vi "CN Config Panel.vi"(8 "error in":errorcluster, 11 "Path":path) -> (0 "error out":errorcluster)   [LabVIEW 2014]
uses:
  Type'def/CN Config Ctr.ctl
panel:
  in  "Exit":bool
  in  "Save Data":bool
  in  "CN Configs":T1[](array[typedef])
  # "Customer Information Config"
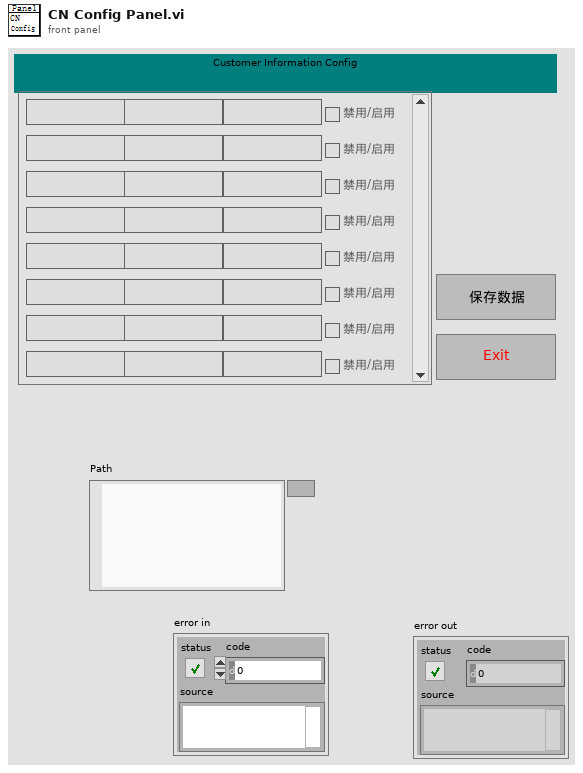
[diagram p1: front panel]
types:
  T1 = typedef "CN Config Ctr.ctl" = cluster{"Model":string, "Pic_Name":string, "CarName":string, "En/Disable":bool}
  T2 = cluster{"Path":path, "CN Configs":T1[], "error in":errorcluster, "Tip":cluster{"info":string, "State":bool}}
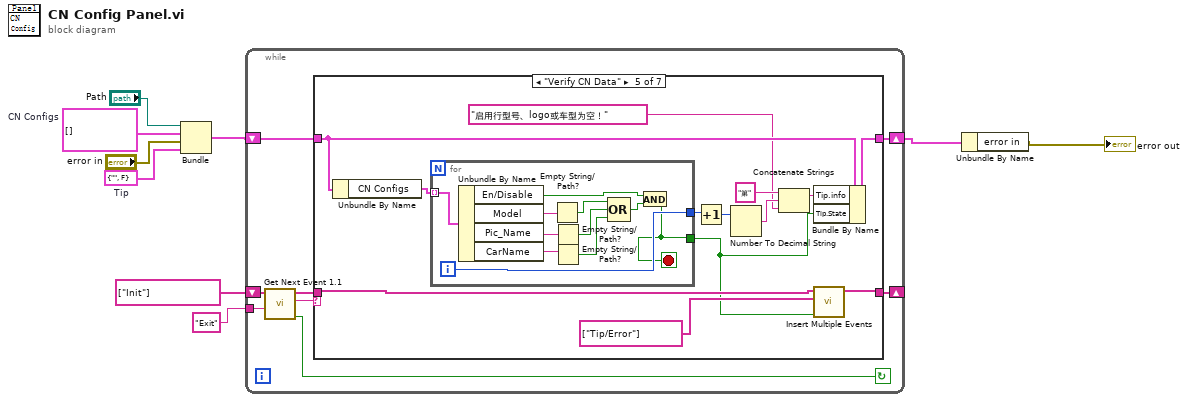
[diagram p0: block diagram]
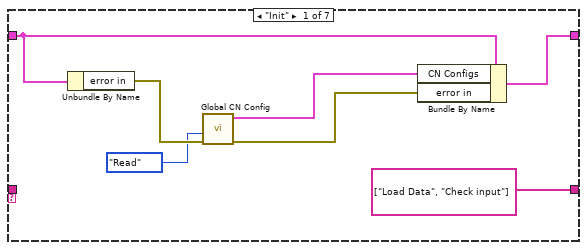
[diagram p2: hidden frame]
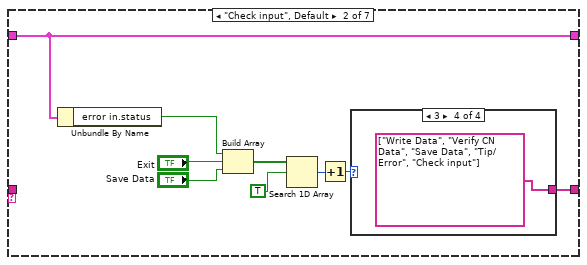
[diagram p3: hidden frame]
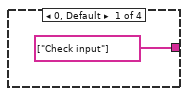
[diagram p4: hidden frame]
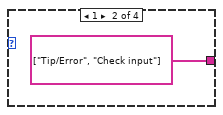
[diagram p5: hidden frame]
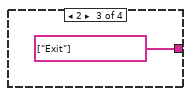
[diagram p6: hidden frame]
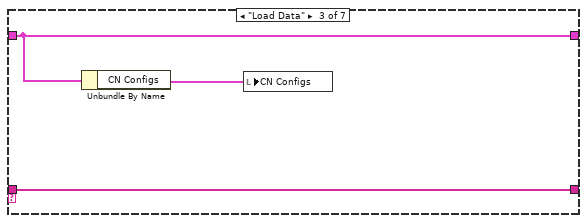
[diagram p7: hidden frame]
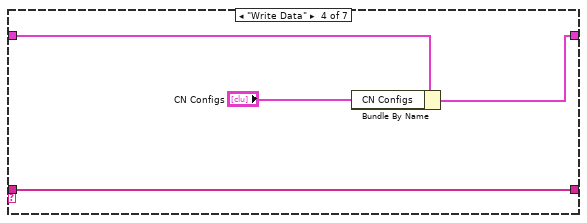
[diagram p8: hidden frame]
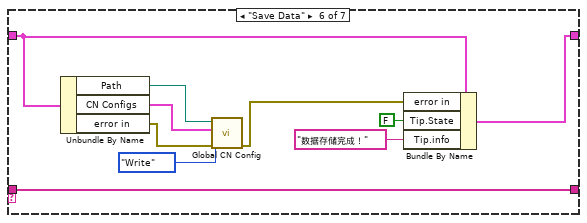
[diagram p9: hidden frame]
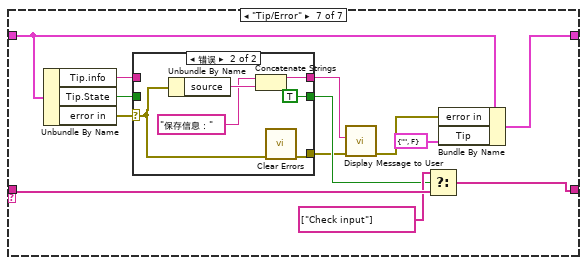
[diagram p10: hidden frame]
diagram:
  w3 = cluster{"info":string, "State":bool} {"info"="", "State"=FALSE}  # Tip
  w7 = T1[] []  # CN Configs
  n1 = Bundle("Path"="Path", "CN Configs"=w7, "error in"="error in", "Tip"=w3) -> (w5:T2)  [unwired: 1 in]
  n2 = while {
    tunnel: "Exit" -> [w14]
    shift-right: [w10] -> _
    shift-left: string[] ["Init"] -> [w15]
    shift-right: [w11] -> w2
    shift-left: w5 -> [w12]
    stop <- w16 continue-if-true
    n3 = call "Get Next Event 1.1.vi"("Exit Event"=w14, "event queue in"=w15) -> ("Condition (Exit:F)"=w16:bool, "next event"=w17:string, "event queue out"=w13:string[])  [unwired: 6 in, 1 out]
    n4 = case shown="\"Verify CN Data\"" w17 {
      tunnel: w13 -> [_ _ w40 w44 w55 w72 w91]
      tunnel: w12 -> [w22 w29 w38 w43 w49 w74 w88]
      tunnel: [w21 w29 w38 w41 w48 w73 w87] -> w11
      tunnel: [string[] ["Load Data", "Check input"] w27 w40 w44 w56 w72 w90] -> w10
      frame "Init" {
        n5 = Unbundle By Name(w22) -> ("error in"=w24:errorcluster)
        n6 = call "Global CN Config.vi"("error in (no error)"=w24, "Mode"=enum16{"Init", "Read", "Write"}."Read") -> ("error out"=w20:errorcluster, "CN Config out"=w19:T1[])  [unwired: 8 in]
        n7 = Bundle By Name(cluster=w22, "CN Configs"=w19, "error in"=w20) -> (w21:T2)
      }
      frame "Check input", Default {
        n8 = Unbundle By Name(w29) -> ("error in.status"=w28:bool)
        n9 = Build Array(w28, "Exit", "Save Data") -> (w31:bool[])
        n10 = Search 1D Array(1D array=w31, element=TRUE) -> (index of element=w26:i32)  [unwired: 1 in]
        n11 = Increment(x=w26) -> (x+1=w25:i32)
        n12 = case shown="3" w25 {
          tunnel: [string[] ["Check input"] string[] ["Tip/Error", "Check input"] string[] ["Exit"] string[] ["Write Data", "Verify CN Data", "Save Data", "Tip/Error", "Check input"]] -> w27
          frame 0, Default {
          }
          frame 1 {
          }
          frame 2 {
          }
          frame 3 {
          }
        }
      }
      frame "Load Data" {
        n13 = Unbundle By Name(w38) -> ("CN Configs"=w39:T1[])
        n14 = local write "CN Configs"(w39) -> ()
      }
      frame "Write Data" {
        n15 = Bundle By Name(cluster=w43, "CN Configs"="CN Configs") -> (w41:T2)
      }
      frame "Verify CN Data" {
        n16 = Unbundle By Name(w49) -> ("CN Configs"=w57:T1[])
        n17 = for {
          tunnel: w57 -> [w68] mode=indexing
          tunnel: [w58] -> w45
          tunnel: [w61] -> w53
          i -> [w61]
          stop <- w58 stop-if-true
          n18 = Unbundle By Name(w68) -> ("En/Disable"=w59:bool, "Model"=w67:string, "Pic_Name"=w66:string, "CarName"=w65:string)
          n19 = Empty String/Path?(string/path=w67) -> (empty?=w64:bool)
          n20 = Empty String/Path?(string/path=w66) -> (empty?=w63:bool)
          n21 = Empty String/Path?(string/path=w65) -> (empty?=w62:bool)
          n22 = Compound Arithmetic op=OR(w64, w63, w62) -> (w60:bool)
          n23 = And(x=w59, y=w60) -> (x .and. y?=w58:bool)
        }
        n24 = Increment(x=w53) -> (x+1=w52:i32)
        n25 = Number To Decimal String(number=w52) -> (decimal integer string=w47:string)  [unwired: 1 in]
        n26 = Concatenate Strings("第", w47, "启用行型号、logo或车型为空！") -> (w50:string)
        n27 = Bundle By Name(cluster=w49, "Tip.info"=w50, "Tip.State"=w45) -> (w48:T2)
        n28 = call "Insert Multiple Events.vi"("Insert all? (T)"=w45, "Events to Insert"=string[] ["Tip/Error"], "Event queue in"=w55) -> ("Event queue out"=w56:string[])  [unwired: 4 in]
      }
      frame "Save Data" {
        n29 = Unbundle By Name(w74) -> ("Path"=w78:path, "CN Configs"=w77:T1[], "error in"=w76:errorcluster)
        n30 = call "Global CN Config.vi"("error in (no error)"=w76, "Mode"=enum16{"Init", "Read", "Write"}."Write", "CN Config"=w77, "Path"=w78) -> ("error out"=w71:errorcluster)  [unwired: 6 in, 1 out]
        n31 = Bundle By Name(cluster=w74, "error in"=w71, "Tip.State"=FALSE, "Tip.info"="数据存储完成！") -> (w73:T2)
      }
      frame "Tip/Error" {
        n32 = Unbundle By Name(w88) -> ("Tip.info"=w82:string, "Tip.State"=w84:bool, "error in"=w85:errorcluster)
        n33 = case shown="错误" w85 {
          selector: w85 -> [w92 w98]
          tunnel: w84 -> [w94 _]
          tunnel: [w94 TRUE ("State")] -> w83
          tunnel: w82 -> [w93 _]
          tunnel: [w93 w96] -> w81
          tunnel: [w92 w100] -> w80
          frame No Error {
          }
          frame Error {
            n34 = Unbundle By Name(w98) -> ("source"=w97:string)
            n35 = Concatenate Strings("保存信息：", w97) -> (w96:string)
            n36 = call <vilib>:"Clear Errors.vi"("error in (no error)"=w98) -> ("error out"=w100:errorcluster)  [unwired: 5 in, 1 out]
          }
        }
        n37 = call "Display Message to User"("error in (no error)"=w80, "Message"=w81) -> ("error out"=w86:errorcluster)  [unwired: 8 in, 1 out]
        n38 = Select(t=string[] ["Check input"], s=w83, f=w91) -> (s? t:f=w90:string[])
        n39 = Bundle By Name(cluster=w88, "error in"=w86, "Tip"=cluster{"info":string, "State":bool} {"info"="", "State"=FALSE}) -> (w87:T2)
      }
    }
  }
  n40 = Unbundle By Name(w2) -> ("error in"=→"error out":errorcluster)
